vi "Flag Finder.vi"(4 "read buffer":string) -> (1 "Output Array":string[](array[string]))   [LabVIEW 2014]
panel:
  out "Boolean":bool
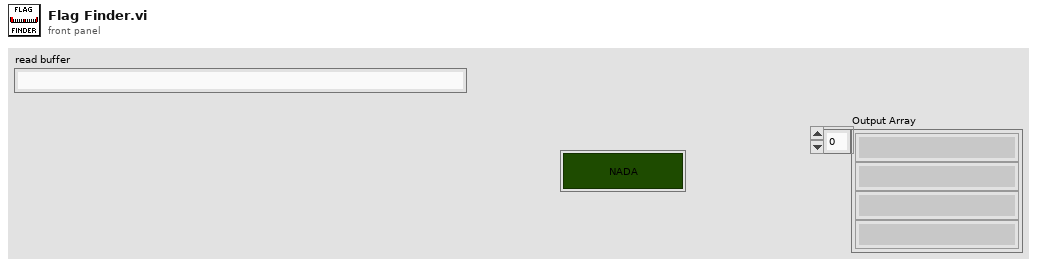
[diagram p1: front panel]
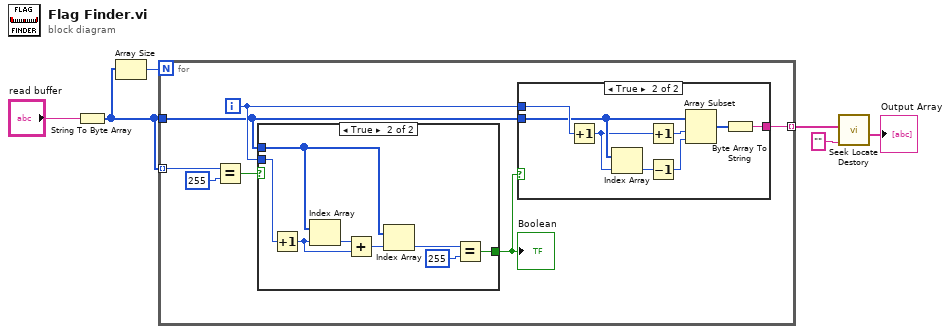
[diagram p0: block diagram]
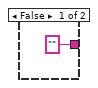
[diagram p2: hidden frame]
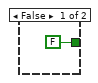
[diagram p3: hidden frame]
diagram:
  n1 = String To Byte Array(string="read buffer") -> (unsigned byte array=w4:u8[])
  n2 = Array Size(array=w4) -> (size(s)=w6:i32)
  n3 = for {
    N: w6 -> [_]
    tunnel: w4 -> [w11] mode=indexing
    tunnel: w4 -> [w8]
    tunnel: [w7] -> w3 mode=indexing
    i -> [w9]
    n4 = Equal?(x=w11, y=u8 255) -> (x = y?=w12:bool)
    n5 = case shown="True" w12 {
      tunnel: w9 -> [_ w29]
      tunnel: w8 -> [_ w31]
      tunnel: [FALSE w25] -> w10
      frame False {
      }
      frame True {
        n6 = Increment(x=w29) -> (x+1=w28:i32)
        n7 = Index Array(array=w31, index=w28) -> (element=w30:u8)
        n8 = Add(x=w30, y=w28) -> (x+y=w24:i32)
        n9 = Index Array(array=w31, index=w24) -> (element=w27:u8)
        n10 = Equal?(x=w27, y=u8 255) -> (x = y?=w25:bool)
      }
    }
    "Boolean" <- w10
    n11 = case shown="True" w10 {
      tunnel: w9 -> [_ w22]
      tunnel: w8 -> [_ w21]
      tunnel: ["" ("string") w19] -> w7
      frame False {
      }
      frame True {
        n12 = Increment(x=w22) -> (x+1=w18:i32)
        n13 = Index Array(array=w21, index=w18) -> (element=w16:u8)
        n14 = Increment(x=w18) -> (x+1=w17:i32)
        n15 = Decrement(x=w16) -> (x-1=w15:u8)
        n16 = Array Subset(array=w21, index=w17, length=w15) -> (w20:u8[])
        n17 = Byte Array To String(unsigned byte array=w20) -> (string=w19:string)
      }
    }
  }
  n18 = call "Seek Locate Destory.vi"("String to Delete"="", "Input String Array"=w3) -> ("Output Array"=→"Output Array":string[])  [unwired: 9 in]
